vi "Frame.Create.vi"(7 "Type":T1, 8 "error in (no error)":errorcluster, 10 "Frame":T3 {"Signals"."Byte Order" items=["Little Endian", "Big Endian"]; "Signals"."Data Type" items=["Signed", "Unsigned", "IEEE Float"]}, 11 "Section Ptr":T2 format="%.0x") -> (0 "error out":errorcluster, 3 "Parent Ref out":T2 format="%.0x")   [LabVIEW 2015, in "Diagnostics Addon System Explorer.lvlib"]
uses:
  Diagnostics Addon System Explorer.lvlib
  Types/Frame.Export.ctl
  Shared/Types/Signal.ctl
  <vilib>/NI Veristand/Custom Device API/Custom Device Item Ref.ctl
  Shared/Types/Type.ctl
  Types/FG.Action.ctl
  <vilib>/NI Veristand/Custom Device API/NI VeriStand - Get Item Property.vi
  <vilib>/NI Veristand/Custom Device API/Get Item Property (U32).vi
  <vilib>/NI Veristand/Custom Device API/NI VeriStand - Set Item Property.vi
  <vilib>/NI Veristand/Custom Device API/Set Item Property (U32).vi
  Shared/SubVIs/Constants.vi
  <vilib>/NI Veristand/Custom Device API/Custom Device API.lvlib
  Shared/Diagnostics Addon Shared.lvlib
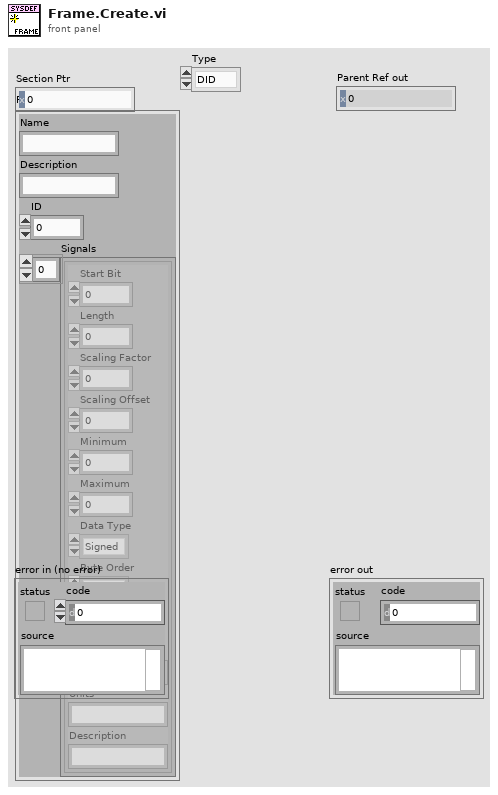
[diagram p1: front panel]
types:
  T1 = typedef "Diagnostics Addon Shared.lvlib/Type.ctl" = enum16{"DID", "CDID", "PID", "CPID", "Read Memory", "Write Memory", "DTC Control", "IO Cmd", "IO Resp", "Routine Start Cmd", "Routine Start Resp", "Routine Request Cmd", "Routine Request Resp", "Routine Stop Cmd", "Routine Stop Resp"}
  T2 = typedef "Custom Device API.lvlib/Custom Device Item Ref.ctl" = u64
  T3 = typedef "Diagnostics Addon System Explorer.lvlib/Frame.Export.ctl" = cluster{"Name":string, "Description":string, "ID":u32, "Signals":T4[]}
  T4 = typedef "Diagnostics Addon Shared.lvlib/Signal.ctl" = cluster{"Start Bit":u8, "Length":u8, "Scaling Factor":dbl, "Scaling Offset":dbl, "Minimum":dbl, "Maximum":dbl, "Data Type":u32, "Byte Order":u32, "Default Value":dbl, "Name":string, "Units":string, "Description":string}
  T5 = typedef "Diagnostics Addon System Explorer.lvlib/FG.Action.ctl" = enum16{"Get", "Set"}
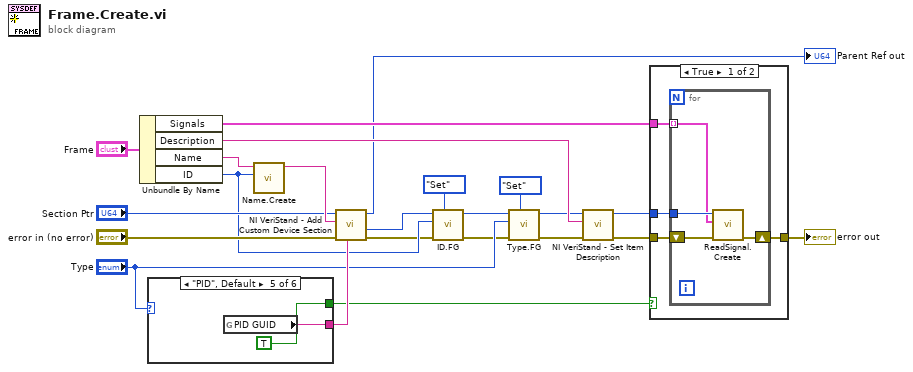
[diagram p0: block diagram]
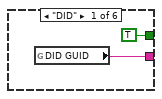
[diagram p2: hidden frame]
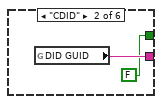
[diagram p3: hidden frame]
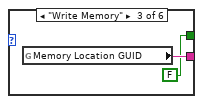
[diagram p4: hidden frame]
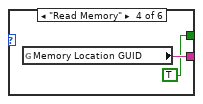
[diagram p5: hidden frame]
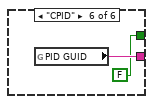
[diagram p6: hidden frame]
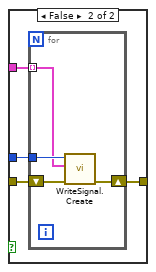
[diagram p7: hidden frame]
diagram:
  n1 = Unbundle By Name("Frame") -> ("Signals"=w22:T4[], "Description"=w14:string, "Name"=w9:string, "ID"=w11:u32)
  n2 = case shown="\"PID\", Default" "Type" {
    tunnel: [w25 w27 w29 w31 w33 w35] -> w19
    tunnel: [TRUE FALSE FALSE TRUE TRUE FALSE] -> w8
    frame "DID" {
      n3 = global read "Constants.vi" "DID GUID"() -> (w25:string)
    }
    frame "CDID" {
      n4 = global read "Constants.vi" "DID GUID"() -> (w27:string)
    }
    frame "Write Memory" {
      n5 = global read "Constants.vi" "Memory Location GUID"() -> (w29:string)
    }
    frame "Read Memory" {
      n6 = global read "Constants.vi" "Memory Location GUID"() -> (w31:string)
    }
    frame "PID", Default {
      n7 = global read "Constants.vi" "PID GUID"() -> (w33:string)
    }
    frame "CPID" {
      n8 = global read "Constants.vi" "PID GUID"() -> (w35:string)
    }
  }
  n9 = call "Name.Create.vi"("PID Number"=w11, "PID Name"=w9) -> ("VS Name"=w23:string)  [unwired: 9 in]
  n10 = call <vilib>:"NI VeriStand - Add Custom Device Section.vi"("GUID (Default Section)"=w19, "error in (no error)"="error in (no error)", "Section Name"=w23, "Parent Ref in"="Section Ptr") -> ("error out"=w5:errorcluster, "Section Ptr"=w6:T2, "Parent Ref out"=→"Parent Ref out":T2)  [unwired: 4 in, 1 out]
  n11 = call "ID.FG.vi"("Action"=FG.Action."Set", "error in (no error)"=w5, "ID"=w11, "Device Item Ref in"=w6) -> ("error out"=w4:errorcluster, "Device Item Ref out"=w3:T2)  [unwired: 5 in, 1 out]
  n12 = call "Type.FG.vi"("Action"=FG.Action."Set", "error in (no error)"=w4, "Type"="Type", "Device Item Ref in"=w3) -> ("error out"=w1:errorcluster, "Device Item Ref out"=w2:T2)  [unwired: 5 in, 1 out]
  n13 = call <vilib>:"NI VeriStand - Set Item Description.vi"("error in (no error)"=w1, "Description"=w14, "Item Ref in"=w2) -> ("error out"=w18:errorcluster, "Item Ref out"=w17:T2)  [unwired: 6 in, 1 out]
  n14 = case shown="True" w8 {
    tunnel: w17 -> [w39 w47]
    tunnel: w22 -> [w38 w46]
    tunnel: [w37 w45] -> w21
    tunnel: w18 -> [w36 w44]
    frame True {
      n15 = for {
        shift-right: [w42] -> w37
        shift-left: w36 -> [w43]
        tunnel: w38 -> [w40] mode=indexing
        tunnel: w39 -> [w41]
        n16 = call "ReadSignal.Create.vi"("error in (no error)"=w43, "Signal Parameters"=w40, "Section Ptr"=w41) -> ("error out"=w42:errorcluster)  [unwired: 7 in, 1 out]
      }
    }
    frame False {
      n17 = for {
        shift-right: [w48] -> w45
        shift-left: w44 -> [w50]
        tunnel: w46 -> [w49] mode=indexing
        tunnel: w47 -> [w51]
        n18 = call "WriteSignal.Create.vi"("error in (no error)"=w50, "Signal Parameters"=w49, "Section Ptr"=w51) -> ("error out"=w48:errorcluster)  [unwired: 7 in, 1 out]
      }
    }
  }
  "error out" <- w21
